vi "getEndEventValue.vi"(8 "error in (no error)":errorcluster, 11 "RampEvent in":refnum<class "RampEvent.lvclass">) -> (0 "error out":errorcluster, 2 "newValue":string, 3 "RampEvent out":refnum<class "RampEvent.lvclass">)   [LabVIEW 2011, in "Tools.lvlib" / "Scripting.lvlib" / "RampEvent.lvclass"]
uses:
  RampEvent.lvclass
  RampEvent.lvclass/RampEvent.ctl
  ScriptEvent.lvclass
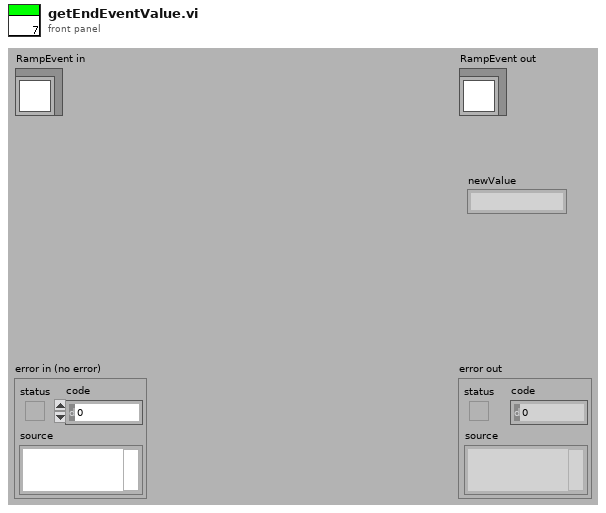
[diagram p1: front panel]
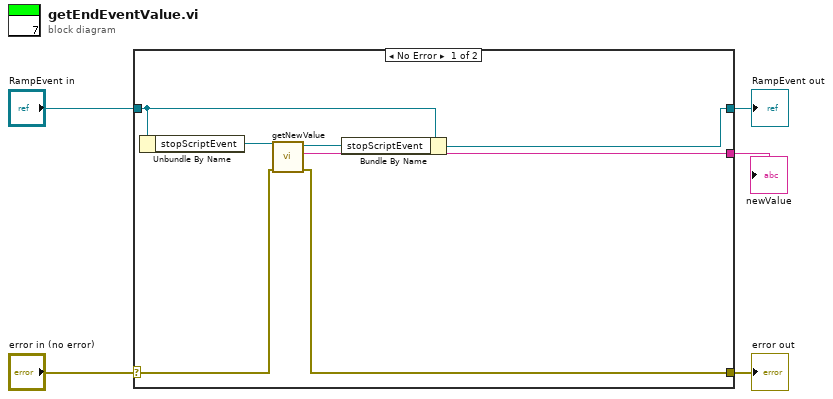
[diagram p0: block diagram]
diagram:
  n1 = case shown="No Error" "error in (no error)" {
    selector: "error in (no error)" -> [w11 w14]
    tunnel: [w6 w14] -> w4
    tunnel: [w8 w13] -> w2
    tunnel: "RampEvent in" -> [w9 w13]
    tunnel: [w10 _] -> w1
    frame No Error {
      n2 = Unbundle By Name(w9) -> ("stopScriptEvent"=w12:refnum<class "ScriptEvent.lvclass">)
      n3 = call "getNewValue.vi"("error in (no error)"=w11, "ScriptEvent.lvclass in"=w12) -> ("error out"=w6:errorcluster, "newValue"=w10:string, "ScriptEvent.lvclass out"=w7:refnum<class "ScriptEvent.lvclass">)  [unwired: 7 in]
      n4 = Bundle By Name(cluster=w9, "stopScriptEvent"=w7) -> (w8:refnum<class "RampEvent.lvclass">)
    }
    frame Error {
    }
  }
  "error out" <- w4
  "RampEvent out" <- w2
  "newValue" <- w1
